vi "Run.vi"(8 "error in (no error)":errorcluster, 11 "Readout Charact in":refnum<class "Readout Charact.lvclass">) -> (0 "error out":errorcluster, 3 "Readout Charact out":refnum<class "Readout Charact.lvclass">)   [LabVIEW 2018, in "Readout Charact.lvclass"]
uses:
  Readout Charact.lvclass
  State Machine/State Machine.lvclass
  Interface/Interface.lvclass
  CCDCamera/CCDCamera.lvclass
  Sync Box/Sync Box.lvclass
  Kinetic Acquisition Mode/Kinetic Acquisition Mode.lvclass
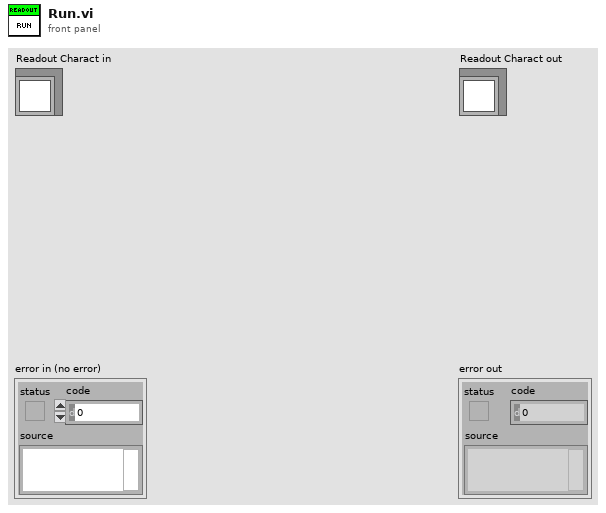
[diagram p1: front panel]
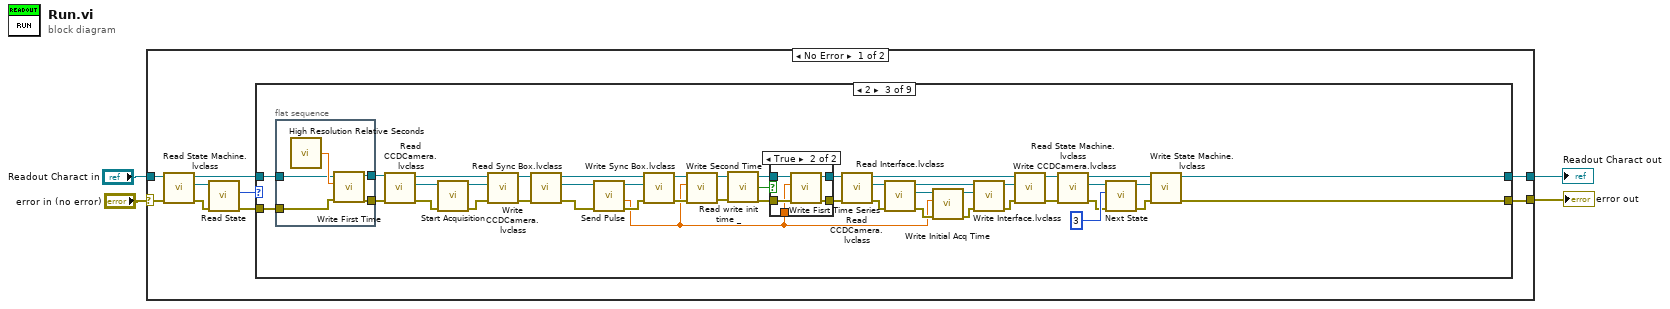
[diagram p0: block diagram]
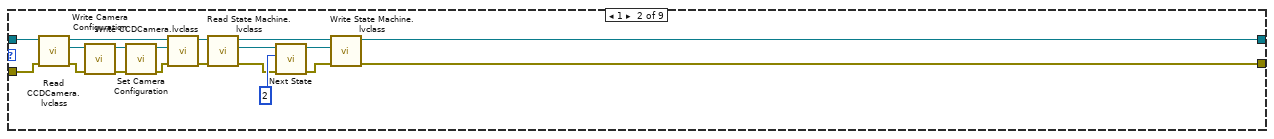
[diagram p3: hidden frame]
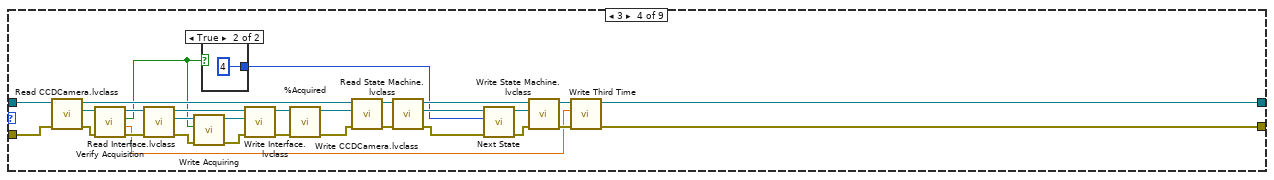
[diagram p5: hidden frame]
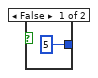
[diagram p6: hidden frame]
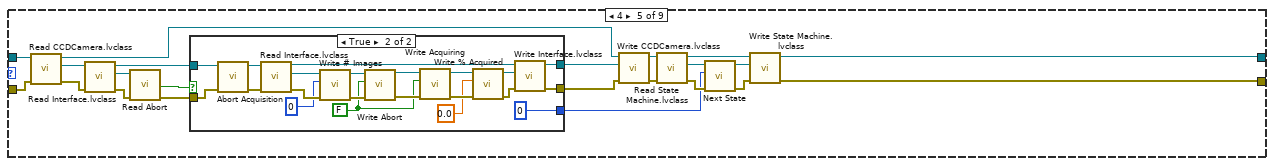
[diagram p7: hidden frame]
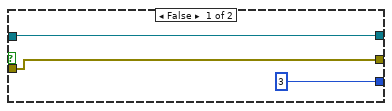
[diagram p8: hidden frame]
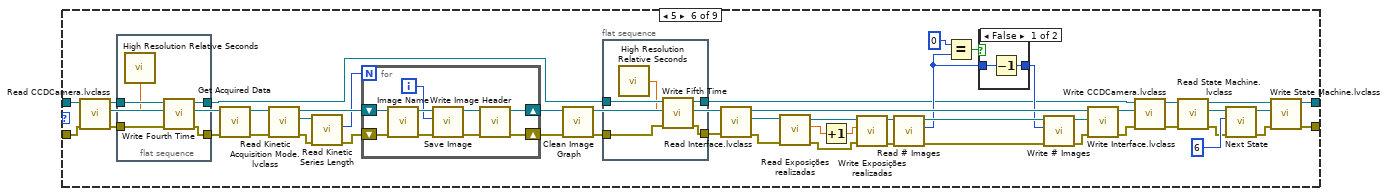
[diagram p9: hidden frame]
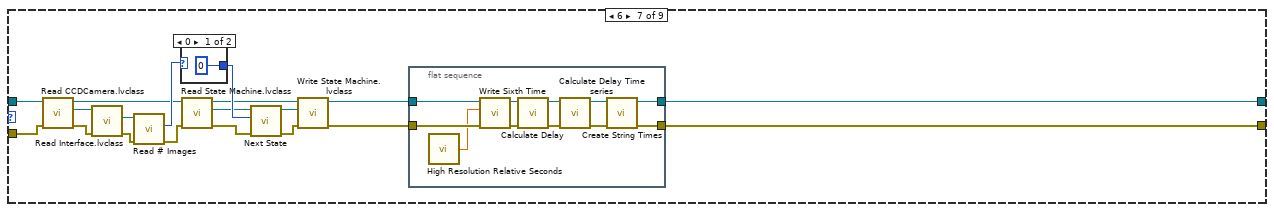
[diagram p11: hidden frame]
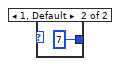
[diagram p12: hidden frame]
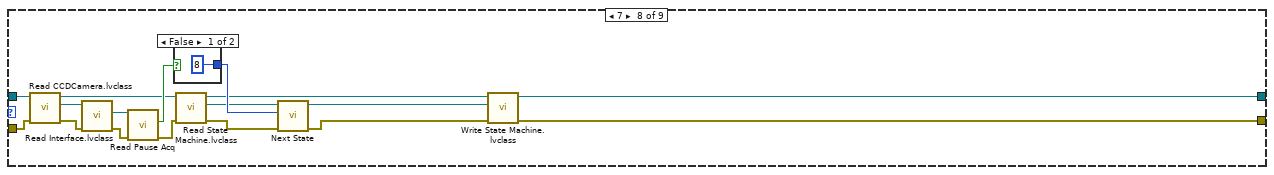
[diagram p13: hidden frame]
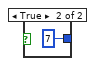
[diagram p14: hidden frame]
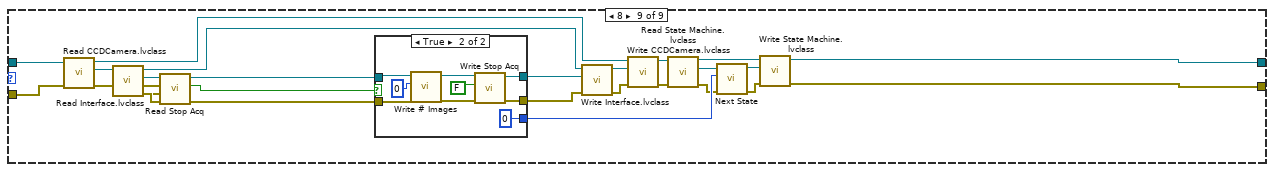
[diagram p15: hidden frame]
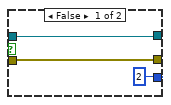
[diagram p16: hidden frame]
diagram:
  n1 = case shown="No Error" "error in (no error)" {
    selector: "error in (no error)" -> [w9 w331]
    tunnel: [w5 w331] -> w3
    tunnel: [w6 w330] -> w1
    tunnel: "Readout Charact in" -> [w8 w330]
    frame No Error {
      n2 = call-dynamic "Read State Machine.lvclass.vi"("error in (no error)"=w9, "Readout Charact in"=w8) -> ("error out"=w10:errorcluster, "State Machine.lvclass"=w11:refnum<class "State Machine.lvclass">, "Readout Charact out"=w7:refnum<class "Readout Charact.lvclass">)  [unwired: 7 in]
      n3 = call-dynamic "Read State.vi"("error in (no error)"=w10, "State Machine in"=w11) -> ("error out"=w12:errorcluster, "State"=w13:u8)  [unwired: 7 in, 1 out]
      n4 = case shown="2" w13 {
        tunnel: w12 -> [w14 w33 w35 w107 w138 w200 w253 w287 w309]
        tunnel: [w15 w17 w71 w94 w126 w189 w243 w275 w293] -> w6
        tunnel: [w14 w16 w70 w95 w125 w188 w242 w274 w294] -> w5
        tunnel: w7 -> [w15 w34 w38 w108 w139 w201 w254 w288 w308]
        frame 0, Default {
        }
        frame 1 {
          n5 = call-dynamic "Read CCDCamera.lvclass.vi"("error in (no error)"=w33, "Readout Charact in"=w34) -> ("error out"=w31:errorcluster, "CCDCamera.lvclass"=w32:refnum<class "CCDCamera.lvclass">, "Readout Charact out"=w26:refnum<class "Readout Charact.lvclass">)  [unwired: 7 in]
          n6 = call-dynamic "Write Camera Configuration.vi"("error in (no error)"=w31, "CCDCamera in"=w32) -> ("error out"=w29:errorcluster, "CCDCamera out"=w30:refnum<class "CCDCamera.lvclass">)  [unwired: 8 in]
          n7 = call "Set Camera Configuration.vi"("error in (no error)"=w29, "CCDCamera in"=w30) -> ("error out"=w28:errorcluster, "CCDCamera out"=w27:refnum<class "CCDCamera.lvclass">)  [unwired: 8 in]
          n8 = call-dynamic "Write CCDCamera.lvclass.vi"("error in (no error)"=w28, "CCDCamera.lvclass"=w27, "Readout Charact in"=w26) -> ("error out"=w25:errorcluster, "Readout Charact out"=w24:refnum<class "Readout Charact.lvclass">)  [unwired: 7 in]
          n9 = call-dynamic "Read State Machine.lvclass.vi"("error in (no error)"=w25, "Readout Charact in"=w24) -> ("error out"=w22:errorcluster, "State Machine.lvclass"=w21:refnum<class "State Machine.lvclass">, "Readout Charact out"=w18:refnum<class "Readout Charact.lvclass">)  [unwired: 7 in]
          n10 = call "Next State.vi"("error in (no error)"=w22, "New_State"=2, "State Machine in"=w21) -> ("error out"=w20:errorcluster, "State Machine out"=w19:refnum<class "State Machine.lvclass">)  [unwired: 7 in]
          n11 = call-dynamic "Write State Machine.lvclass.vi"("error in (no error)"=w20, "State Machine.lvclass"=w19, "Readout Charact in"=w18) -> ("error out"=w16:errorcluster, "Readout Charact out"=w17:refnum<class "Readout Charact.lvclass">)  [unwired: 7 in]
        }
        frame 2 {
          n12 = flat-sequence {
            tunnel: w38 -> [w84]
            tunnel: [w83] -> w37
            tunnel: [w82] -> w36
            tunnel: w35 -> [w81]
            frame #0 {
              n13 = call <vilib>:"High Resolution Relative Seconds.vi"() -> ("relative seconds"=w85:dbl)
              n14 = call-dynamic "Write First Time.vi"("error in (no error)"=w81, "First Time"=w85, "Readout Charact in"=w84) -> ("error out"=w82:errorcluster, "Readout Charact out"=w83:refnum<class "Readout Charact.lvclass">)  [unwired: 7 in]
            }
          }
          n15 = call-dynamic "Read CCDCamera.lvclass.vi"("error in (no error)"=w36, "Readout Charact in"=w37) -> ("error out"=w80:errorcluster, "CCDCamera.lvclass"=w79:refnum<class "CCDCamera.lvclass">, "Readout Charact out"=w78:refnum<class "Readout Charact.lvclass">)  [unwired: 7 in]
          n16 = call "Start Acquisition.vi"("error in (no error)"=w80, "CCDCamera in"=w79) -> ("error out"=w45:errorcluster, "CCDCamera out"=w44:refnum<class "CCDCamera.lvclass">)  [unwired: 8 in]
          n17 = call-dynamic "Write CCDCamera.lvclass.vi"("error in (no error)"=w45, "CCDCamera.lvclass"=w44, "Readout Charact in"=w78) -> ("error out"=w68:errorcluster, "Readout Charact out"=w69:refnum<class "Readout Charact.lvclass">)  [unwired: 7 in]
          n18 = call-dynamic "Read Sync Box.lvclass.vi"("error in (no error)"=w68, "Readout Charact in"=w69) -> ("error out"=w66:errorcluster, "Sync Box.lvclass"=w67:refnum<class "Sync Box.lvclass">, "Readout Charact out"=w63:refnum<class "Readout Charact.lvclass">)  [unwired: 7 in]
          n19 = call "Send Pulse.vi"("error in (no error)"=w66, "Sync Box in"=w67) -> ("error out"=w64:errorcluster, "Init acquisition time"=w39:dbl, "Sync Box out"=w65:refnum<class "Sync Box.lvclass">)  [unwired: 7 in]
          n20 = call-dynamic "Write Sync Box.lvclass.vi"("error in (no error)"=w64, "Sync Box.lvclass"=w65, "Readout Charact in"=w63) -> ("error out"=w43:errorcluster, "Readout Charact out"=w42:refnum<class "Readout Charact.lvclass">)  [unwired: 7 in]
          n21 = call-dynamic "Write Second Time.vi"("error in (no error)"=w43, "Second Time"=w39, "Readout Charact in"=w42) -> ("error out"=w40:errorcluster, "Readout Charact out"=w41:refnum<class "Readout Charact.lvclass">)  [unwired: 7 in]
          n22 = call-dynamic "Read write init time _.vi"("error in (no error)"=w40, "Readout Charact in"=w41) -> ("error out"=w50:errorcluster, "write init time ?"=w46:bool, "Readout Charact out"=w49:refnum<class "Readout Charact.lvclass">)  [unwired: 7 in]
          n23 = case shown="True" w46 {
            tunnel: w50 -> [w86 w89]
            tunnel: w49 -> [w87 w90]
            tunnel: [w87 w91] -> w48
            tunnel: [w86 w92] -> w47
            tunnel: w39 -> [_ w88]
            frame False {
            }
            frame True {
              n24 = call-dynamic "Write Fisrt Time Series.vi"("error in (no error)"=w89, "Fisrt Time Series"=w88, "Readout Charact in"=w90) -> ("error out"=w92:errorcluster, "Readout Charact out"=w91:refnum<class "Readout Charact.lvclass">)  [unwired: 7 in]
            }
          }
          n25 = call-dynamic "Read CCDCamera.lvclass.vi"("error in (no error)"=w47, "Readout Charact in"=w48) -> ("error out"=w62:errorcluster, "CCDCamera.lvclass"=w61:refnum<class "CCDCamera.lvclass">, "Readout Charact out"=w53:refnum<class "Readout Charact.lvclass">)  [unwired: 7 in]
          n26 = call-dynamic "Read Interface.lvclass.vi"("error in (no error)"=w62, "CCDCamera in"=w61) -> ("error out"=w59:errorcluster, "Interface.lvclass"=w60:refnum<class "Interface.lvclass">, "CCDCamera out"=w56:refnum<class "CCDCamera.lvclass">)  [unwired: 7 in]
          n27 = call-dynamic "Write Initial Acq Time.vi"("error in (no error)"=w59, "Initial Acq Time"=w39, "Interface in"=w60) -> ("error out"=w57:errorcluster, "Interface out"=w58:refnum<class "Interface.lvclass">)  [unwired: 7 in]
          n28 = call-dynamic "Write Interface.lvclass.vi"("error in (no error)"=w57, "Interface.lvclass"=w58, "CCDCamera in"=w56) -> ("error out"=w55:errorcluster, "CCDCamera out"=w54:refnum<class "CCDCamera.lvclass">)  [unwired: 7 in]
          n29 = call-dynamic "Write CCDCamera.lvclass.vi"("error in (no error)"=w55, "CCDCamera.lvclass"=w54, "Readout Charact in"=w53) -> ("error out"=w51:errorcluster, "Readout Charact out"=w52:refnum<class "Readout Charact.lvclass">)  [unwired: 7 in]
          n30 = call-dynamic "Read State Machine.lvclass.vi"("error in (no error)"=w51, "Readout Charact in"=w52) -> ("error out"=w76:errorcluster, "State Machine.lvclass"=w75:refnum<class "State Machine.lvclass">, "Readout Charact out"=w72:refnum<class "Readout Charact.lvclass">)  [unwired: 7 in]
          n31 = call "Next State.vi"("error in (no error)"=w76, "New_State"=3, "State Machine in"=w75) -> ("error out"=w74:errorcluster, "State Machine out"=w73:refnum<class "State Machine.lvclass">)  [unwired: 7 in]
          n32 = call-dynamic "Write State Machine.lvclass.vi"("error in (no error)"=w74, "State Machine.lvclass"=w73, "Readout Charact in"=w72) -> ("error out"=w70:errorcluster, "Readout Charact out"=w71:refnum<class "Readout Charact.lvclass">)  [unwired: 7 in]
        }
        frame 3 {
          n33 = call-dynamic "Read CCDCamera.lvclass.vi"("error in (no error)"=w107, "Readout Charact in"=w108) -> ("error out"=w109:errorcluster, "CCDCamera.lvclass"=w110:refnum<class "CCDCamera.lvclass">, "Readout Charact out"=w111:refnum<class "Readout Charact.lvclass">)  [unwired: 7 in]
          n34 = call "Verify Acquisition.vi"("error in (no error)"=w109, "CCDCamera in"=w110) -> ("error out"=w122:errorcluster, "time end acq"=w93:dbl, "Acquiring"=w98:bool, "CCDCamera out"=w121:refnum<class "CCDCamera.lvclass">)  [unwired: 6 in]
          n35 = call-dynamic "Read Interface.lvclass.vi"("error in (no error)"=w122, "CCDCamera in"=w121) -> ("error out"=w114:errorcluster, "Interface.lvclass"=w115:refnum<class "Interface.lvclass">, "CCDCamera out"=w118:refnum<class "CCDCamera.lvclass">)  [unwired: 7 in]
          n36 = call-dynamic "Write Acquiring.vi"("error in (no error)"=w114, "Acquiring"=w98, "Interface in"=w115) -> ("error out"=w120:errorcluster, "Interface out"=w119:refnum<class "Interface.lvclass">)  [unwired: 7 in]
          n37 = case shown="True" w98 {
            tunnel: [u32 5 ("New_State") u32 4 ("New_State")] -> w99
            frame False {
            }
            frame True {
            }
          }
          n38 = call-dynamic "Write Interface.lvclass.vi"("error in (no error)"=w120, "Interface.lvclass"=w119, "CCDCamera in"=w118) -> ("error out"=w117:errorcluster, "CCDCamera out"=w116:refnum<class "CCDCamera.lvclass">)  [unwired: 7 in]
          n39 = call "%Acquired.vi"("error in (no error)"=w117, "CCDCamera in"=w116) -> ("error out"=w113:errorcluster, "CCDCamera out"=w112:refnum<class "CCDCamera.lvclass">)  [unwired: 8 in]
          n40 = call-dynamic "Write CCDCamera.lvclass.vi"("error in (no error)"=w113, "CCDCamera.lvclass"=w112, "Readout Charact in"=w111) -> ("error out"=w101:errorcluster, "Readout Charact out"=w100:refnum<class "Readout Charact.lvclass">)  [unwired: 7 in]
          n41 = call-dynamic "Read State Machine.lvclass.vi"("error in (no error)"=w101, "Readout Charact in"=w100) -> ("error out"=w106:errorcluster, "State Machine.lvclass"=w105:refnum<class "State Machine.lvclass">, "Readout Charact out"=w102:refnum<class "Readout Charact.lvclass">)  [unwired: 7 in]
          n42 = call "Next State.vi"("error in (no error)"=w106, "New_State"=w99, "State Machine in"=w105) -> ("error out"=w104:errorcluster, "State Machine out"=w103:refnum<class "State Machine.lvclass">)  [unwired: 7 in]
          n43 = call-dynamic "Write State Machine.lvclass.vi"("error in (no error)"=w104, "State Machine.lvclass"=w103, "Readout Charact in"=w102) -> ("error out"=w96:errorcluster, "Readout Charact out"=w97:refnum<class "Readout Charact.lvclass">)  [unwired: 7 in]
          n44 = call-dynamic "Write Third Time.vi"("error in (no error)"=w96, "Third Time"=w93, "Readout Charact in"=w97) -> ("error out"=w95:errorcluster, "Readout Charact out"=w94:refnum<class "Readout Charact.lvclass">)  [unwired: 7 in]
        }
        frame 4 {
          n45 = call-dynamic "Read CCDCamera.lvclass.vi"("error in (no error)"=w138, "Readout Charact in"=w139) -> ("error out"=w141:errorcluster, "CCDCamera.lvclass"=w140:refnum<class "CCDCamera.lvclass">, "Readout Charact out"=w130:refnum<class "Readout Charact.lvclass">)  [unwired: 7 in]
          n46 = call-dynamic "Read Interface.lvclass.vi"("error in (no error)"=w141, "CCDCamera in"=w140) -> ("error out"=w144:errorcluster, "Interface.lvclass"=w143:refnum<class "Interface.lvclass">, "CCDCamera out"=w142:refnum<class "CCDCamera.lvclass">)  [unwired: 7 in]
          n47 = call-dynamic "Read Abort.vi"("error in (no error)"=w144, "Interface in"=w143) -> ("error out"=w145:errorcluster, "Abort"=w146:bool)  [unwired: 7 in, 1 out]
          n48 = case shown="True" w146 {
            tunnel: w145 -> [w148 w160]
            tunnel: [3 0] -> w127
            tunnel: w142 -> [w147 w161]
            tunnel: [w148 w159] -> w132
            tunnel: [w147 w158] -> w131
            frame False {
            }
            frame True {
              w151 = FALSE ("Abort")
              n49 = call "Abort Acquisition.vi"("error in (no error)"=w160, "CCDCamera in"=w161) -> ("error out"=w167:errorcluster, "CCDCamera out"=w166:refnum<class "CCDCamera.lvclass">)  [unwired: 8 in]
              n50 = call-dynamic "Read Interface.lvclass.vi"("error in (no error)"=w167, "CCDCamera in"=w166) -> ("error out"=w164:errorcluster, "Interface.lvclass"=w165:refnum<class "Interface.lvclass">, "CCDCamera out"=w163:refnum<class "CCDCamera.lvclass">)  [unwired: 7 in]
              n51 = call-dynamic "Write # Images.vi"("error in (no error)"=w164, "# Images"=u32 0, "Interface in"=w165) -> ("error out"=w169:errorcluster, "Interface out"=w168:refnum<class "Interface.lvclass">)  [unwired: 7 in]
              n52 = call-dynamic "Write Abort.vi"("error in (no error)"=w169, "Abort"=w151, "Interface in"=w168) -> ("error out"=w152:errorcluster, "Interface out"=w155:refnum<class "Interface.lvclass">)  [unwired: 7 in]
              n53 = call-dynamic "Write Acquiring.vi"("error in (no error)"=w152, "Acquiring"=w151, "Interface in"=w155) -> ("error out"=w153:errorcluster, "Interface out"=w154:refnum<class "Interface.lvclass">)  [unwired: 7 in]
              n54 = call-dynamic "Write % Acquired.vi"("error in (no error)"=w153, "% Acquired"=0.0, "Interface in"=w154) -> ("error out"=w156:errorcluster, "Interface out"=w157:refnum<class "Interface.lvclass">)  [unwired: 7 in]
              n55 = call-dynamic "Write Interface.lvclass.vi"("error in (no error)"=w156, "Interface.lvclass"=w157, "CCDCamera in"=w163) -> ("error out"=w159:errorcluster, "CCDCamera out"=w158:refnum<class "CCDCamera.lvclass">)  [unwired: 7 in]
            }
          }
          n56 = call-dynamic "Write CCDCamera.lvclass.vi"("error in (no error)"=w132, "CCDCamera.lvclass"=w131, "Readout Charact in"=w130) -> ("error out"=w128:errorcluster, "Readout Charact out"=w129:refnum<class "Readout Charact.lvclass">)  [unwired: 7 in]
          n57 = call-dynamic "Read State Machine.lvclass.vi"("error in (no error)"=w128, "Readout Charact in"=w129) -> ("error out"=w137:errorcluster, "State Machine.lvclass"=w136:refnum<class "State Machine.lvclass">, "Readout Charact out"=w133:refnum<class "Readout Charact.lvclass">)  [unwired: 7 in]
          n58 = call "Next State.vi"("error in (no error)"=w137, "New_State"=w127, "State Machine in"=w136) -> ("error out"=w135:errorcluster, "State Machine out"=w134:refnum<class "State Machine.lvclass">)  [unwired: 7 in]
          n59 = call-dynamic "Write State Machine.lvclass.vi"("error in (no error)"=w135, "State Machine.lvclass"=w134, "Readout Charact in"=w133) -> ("error out"=w125:errorcluster, "Readout Charact out"=w126:refnum<class "Readout Charact.lvclass">)  [unwired: 7 in]
        }
        frame 5 {
          n60 = call-dynamic "Read CCDCamera.lvclass.vi"("error in (no error)"=w200, "Readout Charact in"=w201) -> ("error out"=w185:errorcluster, "CCDCamera.lvclass"=w202:refnum<class "CCDCamera.lvclass">, "Readout Charact out"=w186:refnum<class "Readout Charact.lvclass">)  [unwired: 7 in]
          n61 = flat-sequence {
            tunnel: [w238] -> w187
            tunnel: [w237] -> w175
            tunnel: w186 -> [w236]
            tunnel: w185 -> [w235]
            frame #0 {
              n62 = call <vilib>:"High Resolution Relative Seconds.vi"() -> ("relative seconds"=w234:dbl)
              n63 = call-dynamic "Write Fourth Time.vi"("error in (no error)"=w235, "Fourth Time"=w234, "Readout Charact in"=w236) -> ("error out"=w238:errorcluster, "Readout Charact out"=w237:refnum<class "Readout Charact.lvclass">)  [unwired: 7 in]
            }
          }
          n64 = call "Get Acquired Data.vi"("error in (no error)"=w187, "CCDCamera in"=w202) -> ("error out"=w177:errorcluster, "CCDCamera out"=w176:refnum<class "CCDCamera.lvclass">)  [unwired: 7 in, 1 out]
          n65 = call-dynamic "Read Kinetic Acquisition Mode.lvclass.vi"("error in (no error)"=w177, "CCDCamera in"=w176) -> ("error out"=w178:errorcluster, "Kinetic Acquisition Mode.lvclass"=w179:refnum<class "Kinetic Acquisition Mode.lvclass">, "CCDCamera out"=w181:refnum<class "CCDCamera.lvclass">)  [unwired: 7 in]
          n66 = call-dynamic "Read Kinetic Series Length.vi"("error in (no error)"=w178, "Kinetic Acquisition Mode in"=w179) -> ("error out"=w182:errorcluster, "Kinetic Series Length"=w180:u32)  [unwired: 7 in, 1 out]
          n67 = for {
            N: w180 -> [_]
            shift-right: [w220] -> w173
            shift-left: w181 -> [w226]
            shift-right: [w221] -> w174
            shift-left: w182 -> [w225]
            i -> [w224]
            n68 = call "Image Name.vi"("error in (no error)"=w225, "CCDCamera in"=w226) -> ("error out"=w227:errorcluster, "CCDCamera out"=w228:refnum<class "CCDCamera.lvclass">)  [unwired: 8 in]
            n69 = call "Save Image.vi"("error in (no error)"=w227, "Shift"=w224, "CCDCamera in"=w228) -> ("error out"=w222:errorcluster, "CCDCamera out"=w223:refnum<class "CCDCamera.lvclass">)  [unwired: 7 in]
            n70 = call "Write Image Header.vi"("error in (no error)"=w222, "CCDCamera in"=w223) -> ("error out"=w221:errorcluster, "CCDCamera out"=w220:refnum<class "CCDCamera.lvclass">)  [unwired: 8 in]
          }
          n71 = call "Clean Image Graph.vi"("error in (no error)"=w174, "CCDCamera in"=w173) -> ("error out"=w171:errorcluster, "CCDCamera out"=w172:refnum<class "CCDCamera.lvclass">)  [unwired: 8 in]
          n72 = flat-sequence {
            tunnel: w171 -> [w231]
            tunnel: [w232] -> w184
            tunnel: w175 -> [w230]
            tunnel: [w233] -> w183
            frame #0 {
              n73 = call <vilib>:"High Resolution Relative Seconds.vi"() -> ("relative seconds"=w229:dbl)
              n74 = call-dynamic "Write Fifth Time.vi"("error in (no error)"=w231, "Fifth Time"=w229, "Readout Charact in"=w230) -> ("error out"=w232:errorcluster, "Readout Charact out"=w233:refnum<class "Readout Charact.lvclass">)  [unwired: 7 in]
            }
          }
          n75 = call-dynamic "Read Interface.lvclass.vi"("error in (no error)"=w184, "CCDCamera in"=w172) -> ("error out"=w213:errorcluster, "Interface.lvclass"=w215:refnum<class "Interface.lvclass">, "CCDCamera out"=w214:refnum<class "CCDCamera.lvclass">)  [unwired: 7 in]
          n76 = call-dynamic "Read Exposições realizadas.vi"("error in (no error)"=w213, "Interface in"=w215) -> ("error out"=w216:errorcluster, "Exposições realizadas"=w219:dbl, "Interface out"=w217:refnum<class "Interface.lvclass">)  [unwired: 7 in]
          n77 = Increment(x=w219) -> (x+1=w218:dbl)
          n78 = call-dynamic "Write Exposições realizadas.vi"("error in (no error)"=w216, "Exposições realizadas"=w218, "Interface in"=w217) -> ("error out"=w212:errorcluster, "Interface out"=w211:refnum<class "Interface.lvclass">)  [unwired: 7 in]
          n79 = call-dynamic "Read # Images.vi"("error in (no error)"=w212, "Interface in"=w211) -> ("error out"=w209:errorcluster, "# Images"=w205:u32, "Interface out"=w210:refnum<class "Interface.lvclass">)  [unwired: 7 in]
          n80 = Equal?(x=u32 0, y=w205) -> (x = y?=w208:bool)
          n81 = case shown="False" w208 {
            tunnel: [w240 w241] -> w206
            tunnel: w205 -> [w239 w241]
            frame False {
              n82 = Decrement(x=w239) -> (x-1=w240:u32)
            }
            frame True {
            }
          }
          n83 = call-dynamic "Write # Images.vi"("error in (no error)"=w209, "# Images"=w206, "Interface in"=w210) -> ("error out"=w203:errorcluster, "Interface out"=w204:refnum<class "Interface.lvclass">)  [unwired: 7 in]
          n84 = call-dynamic "Write Interface.lvclass.vi"("error in (no error)"=w203, "Interface.lvclass"=w204, "CCDCamera in"=w214) -> ("error out"=w199:errorcluster, "CCDCamera out"=w198:refnum<class "CCDCamera.lvclass">)  [unwired: 7 in]
          n85 = call-dynamic "Write CCDCamera.lvclass.vi"("error in (no error)"=w199, "CCDCamera.lvclass"=w198, "Readout Charact in"=w183) -> ("error out"=w191:errorcluster, "Readout Charact out"=w190:refnum<class "Readout Charact.lvclass">)  [unwired: 7 in]
          n86 = call-dynamic "Read State Machine.lvclass.vi"("error in (no error)"=w191, "Readout Charact in"=w190) -> ("error out"=w196:errorcluster, "State Machine.lvclass"=w195:refnum<class "State Machine.lvclass">, "Readout Charact out"=w192:refnum<class "Readout Charact.lvclass">)  [unwired: 7 in]
          n87 = call "Next State.vi"("error in (no error)"=w196, "New_State"=6, "State Machine in"=w195) -> ("error out"=w194:errorcluster, "State Machine out"=w193:refnum<class "State Machine.lvclass">)  [unwired: 7 in]
          n88 = call-dynamic "Write State Machine.lvclass.vi"("error in (no error)"=w194, "State Machine.lvclass"=w193, "Readout Charact in"=w192) -> ("error out"=w188:errorcluster, "Readout Charact out"=w189:refnum<class "Readout Charact.lvclass">)  [unwired: 7 in]
        }
        frame 6 {
          n89 = call-dynamic "Read CCDCamera.lvclass.vi"("error in (no error)"=w253, "Readout Charact in"=w254) -> ("error out"=w256:errorcluster, "CCDCamera.lvclass"=w255:refnum<class "CCDCamera.lvclass">, "Readout Charact out"=w252:refnum<class "Readout Charact.lvclass">)  [unwired: 7 in]
          n90 = call-dynamic "Read Interface.lvclass.vi"("error in (no error)"=w256, "CCDCamera in"=w255) -> ("error out"=w258:errorcluster, "Interface.lvclass"=w257:refnum<class "Interface.lvclass">)  [unwired: 7 in, 1 out]
          n91 = call-dynamic "Read # Images.vi"("error in (no error)"=w258, "Interface in"=w257) -> ("error out"=w251:errorcluster, "# Images"=w259:u32)  [unwired: 7 in, 1 out]
          n92 = case shown="0" w259 {
            tunnel: [u32 0 ("New_State") 7] -> w260
            frame 0 {
            }
            frame 1, Default {
            }
          }
          n93 = call-dynamic "Read State Machine.lvclass.vi"("error in (no error)"=w251, "Readout Charact in"=w252) -> ("error out"=w249:errorcluster, "State Machine.lvclass"=w250:refnum<class "State Machine.lvclass">, "Readout Charact out"=w246:refnum<class "Readout Charact.lvclass">)  [unwired: 7 in]
          n94 = call "Next State.vi"("error in (no error)"=w249, "New_State"=w260, "State Machine in"=w250) -> ("error out"=w248:errorcluster, "State Machine out"=w247:refnum<class "State Machine.lvclass">)  [unwired: 7 in]
          n95 = call-dynamic "Write State Machine.lvclass.vi"("error in (no error)"=w248, "State Machine.lvclass"=w247, "Readout Charact in"=w246) -> ("error out"=w245:errorcluster, "Readout Charact out"=w244:refnum<class "Readout Charact.lvclass">)  [unwired: 7 in]
          n96 = flat-sequence {
            tunnel: w245 -> [w262]
            tunnel: w244 -> [w263]
            tunnel: [w267] -> w243
            tunnel: [w266] -> w242
            frame #0 {
              n97 = call <vilib>:"High Resolution Relative Seconds.vi"() -> ("relative seconds"=w261:dbl)
              n98 = call-dynamic "Write Sixth Time.vi"("error in (no error)"=w262, "Sixth Time"=w261, "Readout Charact in"=w263) -> ("error out"=w265:errorcluster, "Readout Charact out"=w264:refnum<class "Readout Charact.lvclass">)  [unwired: 7 in]
              n99 = call "Calculate Delay.vi"("error in (no error)"=w265, "Readout Charact in"=w264) -> ("error out"=w270:errorcluster, "Readout Charact out"=w271:refnum<class "Readout Charact.lvclass">)  [unwired: 8 in]
              n100 = call "Calculate Delay Time series.vi"("error in (no error)"=w270, "Readout Charact in"=w271) -> ("error out"=w269:errorcluster, "Readout Charact out"=w268:refnum<class "Readout Charact.lvclass">)  [unwired: 8 in]
              n101 = call "Create String Times.vi"("error in (no error)"=w269, "Readout Charact in"=w268) -> ("error out"=w266:errorcluster, "Readout Charact out"=w267:refnum<class "Readout Charact.lvclass">)  [unwired: 8 in]
            }
          }
        }
        frame 7 {
          n102 = call-dynamic "Read CCDCamera.lvclass.vi"("error in (no error)"=w287, "Readout Charact in"=w288) -> ("error out"=w286:errorcluster, "CCDCamera.lvclass"=w285:refnum<class "CCDCamera.lvclass">, "Readout Charact out"=w282:refnum<class "Readout Charact.lvclass">)  [unwired: 7 in]
          n103 = call-dynamic "Read Interface.lvclass.vi"("error in (no error)"=w286, "CCDCamera in"=w285) -> ("error out"=w283:errorcluster, "Interface.lvclass"=w284:refnum<class "Interface.lvclass">)  [unwired: 7 in, 1 out]
          n104 = call-dynamic "Read Pause Acq.vi"("error in (no error)"=w283, "Interface in"=w284) -> ("error out"=w281:errorcluster, "Pause Acq"=w289:bool)  [unwired: 7 in, 1 out]
          n105 = case shown="False" w289 {
            tunnel: [u32 8 ("# Images") u32 7 ("# Images")] -> w290
            frame False {
            }
            frame True {
            }
          }
          n106 = call-dynamic "Read State Machine.lvclass.vi"("error in (no error)"=w281, "Readout Charact in"=w282) -> ("error out"=w279:errorcluster, "State Machine.lvclass"=w280:refnum<class "State Machine.lvclass">, "Readout Charact out"=w276:refnum<class "Readout Charact.lvclass">)  [unwired: 7 in]
          n107 = call "Next State.vi"("error in (no error)"=w279, "New_State"=w290, "State Machine in"=w280) -> ("error out"=w278:errorcluster, "State Machine out"=w277:refnum<class "State Machine.lvclass">)  [unwired: 7 in]
          n108 = call-dynamic "Write State Machine.lvclass.vi"("error in (no error)"=w278, "State Machine.lvclass"=w277, "Readout Charact in"=w276) -> ("error out"=w274:errorcluster, "Readout Charact out"=w275:refnum<class "Readout Charact.lvclass">)  [unwired: 7 in]
        }
        frame 8 {
          n109 = call-dynamic "Read CCDCamera.lvclass.vi"("error in (no error)"=w309, "Readout Charact in"=w308) -> ("error out"=w311:errorcluster, "CCDCamera.lvclass"=w310:refnum<class "CCDCamera.lvclass">, "Readout Charact out"=w300:refnum<class "Readout Charact.lvclass">)  [unwired: 7 in]
          n110 = call-dynamic "Read Interface.lvclass.vi"("error in (no error)"=w311, "CCDCamera in"=w310) -> ("error out"=w313:errorcluster, "Interface.lvclass"=w312:refnum<class "Interface.lvclass">, "CCDCamera out"=w303:refnum<class "CCDCamera.lvclass">)  [unwired: 7 in]
          n111 = call-dynamic "Read Stop Acq.vi"("error in (no error)"=w313, "Interface in"=w312) -> ("error out"=w314:errorcluster, "Stop Acq"=w316:bool, "Interface out"=w315:refnum<class "Interface.lvclass">)  [unwired: 7 in]
          n112 = case shown="True" w316 {
            tunnel: w315 -> [w318 w323]
            tunnel: w314 -> [w319 w324]
            tunnel: [u32 2 ("# Images") u32 0 ("# Images")] -> w317
            tunnel: [w318 w322] -> w305
            tunnel: [w319 w321] -> w304
            frame False {
            }
            frame True {
              n113 = call-dynamic "Write # Images.vi"("error in (no error)"=w324, "# Images"=u32 0, "Interface in"=w323) -> ("error out"=w325:errorcluster, "Interface out"=w326:refnum<class "Interface.lvclass">)  [unwired: 7 in]
              n114 = call-dynamic "Write Stop Acq.vi"("error in (no error)"=w325, "Stop Acq"=FALSE, "Interface in"=w326) -> ("error out"=w321:errorcluster, "Interface out"=w322:refnum<class "Interface.lvclass">)  [unwired: 7 in]
            }
          }
          n115 = call-dynamic "Write Interface.lvclass.vi"("error in (no error)"=w304, "Interface.lvclass"=w305, "CCDCamera in"=w303) -> ("error out"=w302:errorcluster, "CCDCamera out"=w301:refnum<class "CCDCamera.lvclass">)  [unwired: 7 in]
          n116 = call-dynamic "Write CCDCamera.lvclass.vi"("error in (no error)"=w302, "CCDCamera.lvclass"=w301, "Readout Charact in"=w300) -> ("error out"=w298:errorcluster, "Readout Charact out"=w299:refnum<class "Readout Charact.lvclass">)  [unwired: 7 in]
          n117 = call-dynamic "Read State Machine.lvclass.vi"("error in (no error)"=w298, "Readout Charact in"=w299) -> ("error out"=w307:errorcluster, "State Machine.lvclass"=w306:refnum<class "State Machine.lvclass">, "Readout Charact out"=w295:refnum<class "Readout Charact.lvclass">)  [unwired: 7 in]
          n118 = call "Next State.vi"("error in (no error)"=w307, "New_State"=w317, "State Machine in"=w306) -> ("error out"=w297:errorcluster, "State Machine out"=w296:refnum<class "State Machine.lvclass">)  [unwired: 7 in]
          n119 = call-dynamic "Write State Machine.lvclass.vi"("error in (no error)"=w297, "State Machine.lvclass"=w296, "Readout Charact in"=w295) -> ("error out"=w294:errorcluster, "Readout Charact out"=w293:refnum<class "Readout Charact.lvclass">)  [unwired: 7 in]
        }
      }
    }
    frame Error {
    }
  }
  "error out" <- w3
  "Readout Charact out" <- w1
